vi "Motor_speed_controlling_with_PI_v7_openloop.vi"() -> ()   [LabVIEW 2016]
doc: "This example demonstrates how to generate a PWM signal on a single channel using a LINX device."
uses:
  <vilib>/MakerHub/LINX/Public/Peripherals/Analog/Analog Read 1 Chan.vi
  <vilib>/MakerHub/LINX/Public/Peripherals/Digital/Digital Read 1 Chan.vi
  <vilib>/MakerHub/LINX/Public/Peripherals/Digital/Digital Write 1 Chan.vi
  <vilib>/MakerHub/LINX/Public/Peripherals/PWM/PWM Set Duty Cycle 1 Chan.vi
  <vilib>/MakerHub/LINX/Public/Peripherals/Analog/Analog Read N Chans.vi
  <vilib>/MakerHub/LINX/Public/Peripherals/Digital/Digital Read N Chans.vi
  <vilib>/MakerHub/LINX/Public/Peripherals/Digital/Digital Write N Chans.vi
  <vilib>/MakerHub/LINX/Private/Local IO/LinxAnalogRead.vi
  <vilib>/MakerHub/LINX/Public/Utilities/Check Channel.vi
  <vilib>/MakerHub/LINX/Private/Local IO/LinxDigitalRead.vi
  <vilib>/MakerHub/LINX/Private/Local IO/LinxDigitalWrite.vi
  <vilib>/MakerHub/LINX/Public/Utilities/Open Serial.vi
  <vilib>/addons/control/pid/pid.llb/PID (DBL).vi
  <vilib>/MakerHub/LINX/Public/Peripherals/PWM/PWM Set Duty Cycle N Chans.vi
  <vilib>/MakerHub/LINX/Private/Utilties/Generate Error.vi
  <vilib>/MakerHub/LINX/LMH-LINX.lvlib
  <vilib>/addons/control/pid/NI_PID_pid.lvlib
panel:
  out "Loop Rate (Hz)":u32
  out "PWM Signal":dbl(graph)
  in  "Loop Delay(ms)":u32
  out "Motor Voltage":dbl(graph)
  out "PID Screen":dbl(graph)
  in  "Direction":bool
  out "Motor Speed(RPM)":dbl(knob) scale=0.0..80.0
  in  "Encoder Input Pin":u8
  in  "PID gains":T1={"proportional gain (Kc)"=1.0, "integral time (Ti, min)"=0.01, "derivative time (Td, min)"=0.0} {"derivative time (Td, min)" format="%.3f"; "integral time (Ti, min)" format="%.3f"; "proportional gain (Kc)" format="%.3f"}
  in  "Motor Speed":dbl(knob) scale=0.0..80.0
  in  "PWM Output Pin":u8=3
  in  "Stop Button":bool
  in  "Serial Port":refnum<visa-resource-name>
  # "Direction"
  # "Motor Speed Control\n(RPM)"
  # "Motor Speed \n(RPM)"
  # "PID Settings"
  # "Device and Connection\nSettings"
  # "Forward"
  # "e"
  # "Back"
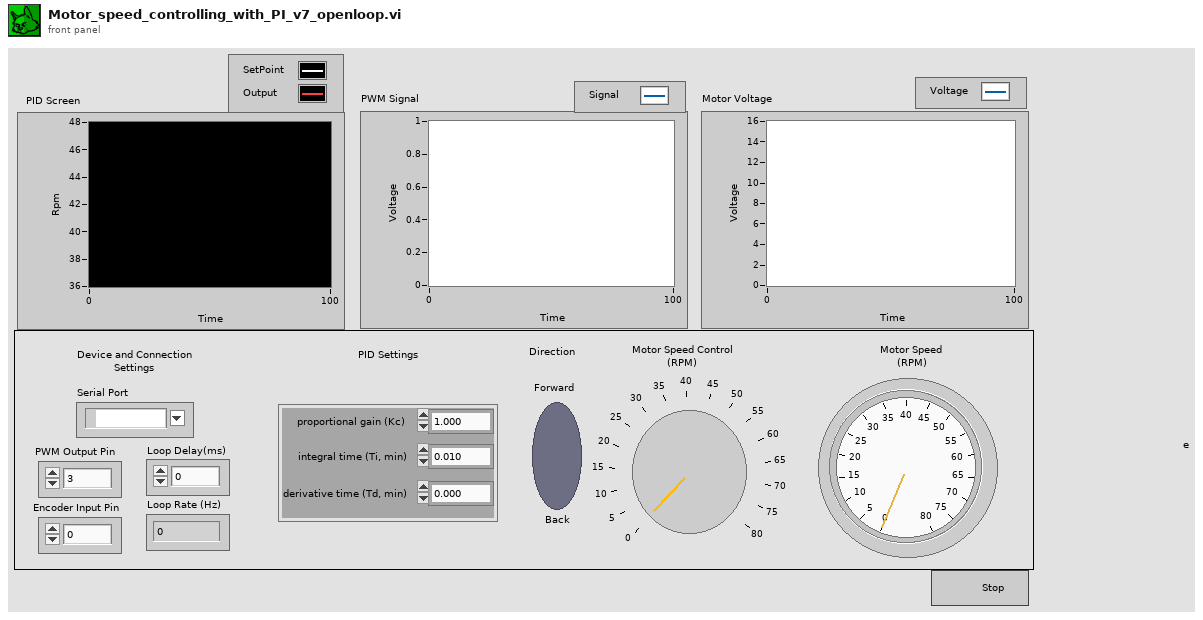
[diagram p1: front panel]
types:
  T1 = cluster{"proportional gain (Kc)":dbl, "integral time (Ti, min)":dbl, "derivative time (Td, min)":dbl}
  T2 = typedef "LMH-LINX.lvlib/LINX Ref.ctl" = cluster{"IO":T3, "Interface":T4, "LINX Device Config":T5}
  T3 = typedef "LMH-LINX.lvlib/Platform.ctl" = enum16{"Remote", "Local"}
  T4 = typedef "LMH-LINX.lvlib/Interface.ctl" = enum16{"Serial", "TCP"}
  T5 = typedef "LMH-LINX.lvlib/Device.lvlib/LINX Device Config.ctl" = cluster{"Interface":T4, "COM Port":refnum<visa-resource-name>, "TCP Configuration":T6, "Device Family":u8, "Device ID":u8, "Device Name":string, "TCP Ref":refnum<k5>, "Channels":T7}
  T6 = typedef "LMH-LINX.lvlib/Device.lvlib/TCP Config.ctl" = cluster{"IP Address":string, "Port":u16}
  T7 = typedef "LMH-LINX.lvlib/Channels.ctl" = cluster{"DI":u8[], "DO":u8[], "AI":u8[], "AO":u8[], "PWM":u8[], "QE":u8[], "UART":u8[], "I2C 2":u8[], "SPI":u8[], "CAN":u8[], "Servo":u8[], "AI Ref (V)":dbl, "AI Resolution (Bits)":u8, "AO Ref (V)":dbl, "AO Resolution (Bits)":u8}
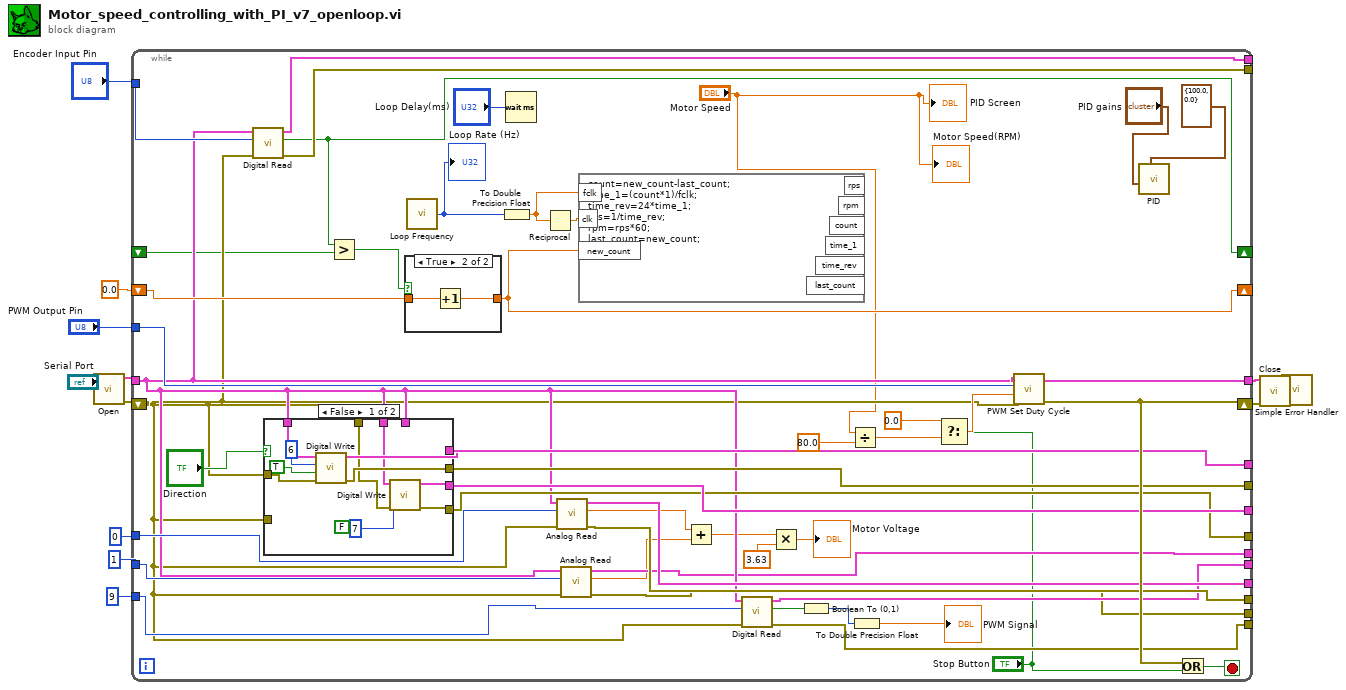
[diagram p0: block diagram]
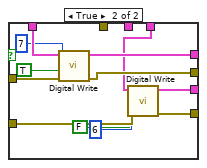
[diagram p3: hidden frame]
diagram:
  n1 = call-poly <vilib>:"Open.vi"("Serial Port"="Serial Port") -> ("Error Out"=w11:errorcluster, "LINX Resource"=w12:T2)  [unwired: 8 in, 1 out]
  n2 = while {
    tunnel: w12 -> [w29]
    tunnel: [w57] -> w10
    shift-right: [w59] -> w9
    shift-left: w11 -> [w28]
    tunnel: "PWM Output Pin" -> [w58]
    tunnel: "Encoder Input Pin" -> [w43]
    tunnel: [w42] -> _
    tunnel: [w41] -> _
    tunnel: [w51] -> _
    tunnel: [w50] -> _
    tunnel: [w47] -> _
    tunnel: [w46] -> _
    tunnel: [w45] -> _
    tunnel: [w44] -> _
    shift-right: [w16] -> _
    shift-left: _ -> [w15]
    shift-right: [w22] -> _
    shift-left: 0.0 -> [w39]
    tunnel: u8 0 ("Analog Channel") -> [w38]
    tunnel: [w37] -> _
    tunnel: [w36] -> _
    tunnel: u8 9 ("Analog Channel") -> [w33]
    tunnel: u8 1 ("Analog Channel") -> [w30]
    tunnel: [w27] -> _
    tunnel: [w26] -> _
    stop <- w60 stop-if-true
    n3 = call-poly <vilib>:"Digital Read.vi"("Error In"=w28, "DI Channel"=w43, "LINX Resource"=w29) -> ("Error Out"=w41:errorcluster, "DI Value"=w16:bool, "LINX Resource"=w42:T2)  [unwired: 6 in]
    n4 = case shown="False" "Direction" {
      tunnel: w29 -> [w75 w87]
      tunnel: w28 -> [w74 w86]
      tunnel: [w73 w84] -> w51
      tunnel: [w72 w83] -> w50
      tunnel: w29 -> [_ w81]
      tunnel: w28 -> [_ w80]
      tunnel: [w67 w79] -> w45
      tunnel: [w66 w78] -> w44
      tunnel: w29 -> [w69 _]
      tunnel: w28 -> [w68 _]
      frame False {
        n5 = call-poly <vilib>:"Digital Write.vi"("Error In"=w74, "Output Value"=TRUE, "DO Channel"=u8 6, "LINX Resource"=w75) -> ("Error Out"=w72:errorcluster, "LINX Resource"=w73:T2)  [unwired: 6 in]
        n6 = call-poly <vilib>:"Digital Write.vi"("Error In"=w68, "Output Value"=FALSE, "DO Channel"=u8 7, "LINX Resource"=w69) -> ("Error Out"=w66:errorcluster, "LINX Resource"=w67:T2)  [unwired: 6 in]
      }
      frame True {
        n7 = call-poly <vilib>:"Digital Write.vi"("Error In"=w86, "Output Value"=TRUE, "DO Channel"=u8 7, "LINX Resource"=w87) -> ("Error Out"=w83:errorcluster, "LINX Resource"=w84:T2)  [unwired: 6 in]
        n8 = call-poly <vilib>:"Digital Write.vi"("Error In"=w80, "Output Value"=FALSE, "DO Channel"=u8 6, "LINX Resource"=w81) -> ("Error Out"=w78:errorcluster, "LINX Resource"=w79:T2)  [unwired: 6 in]
      }
    }
    n9 = Greater?(x=w16, y=w15) -> (0:w14:bool)
    n10 = case shown="True" w14 {
      tunnel: w39 -> [w61 w63]
      tunnel: [w61 w62] -> w22
      frame False {
      }
      frame True {
        n11 = Increment(x=w63) -> (x+1=w62:dbl)
      }
    }
    n12 = call <vilib>:"Loop Frequency.vi"() -> ("Loop Rate (Hz)"=w21:u32)
    "Loop Rate (Hz)" <- w21
    n13 = To Double Precision Float(number=w21) -> (double precision float=w19:dbl)
    n14 = Wait (ms)(milliseconds to wait="Loop Delay(ms)") -> ()  [unwired: 1 out]
    n15 = Reciprocal(x=w19) -> (1/x=w18:dbl)
    n16 = call-poly <vilib>:"Analog Read.vi"("Error In"=w28, "Analog Channel"=w38, "LINX Resource"=w29) -> ("Error Out"=w46:errorcluster, "Voltage"=w25:dbl, "LINX Resource"=w47:T2)  [unwired: 5 in, 1 out]
    n17 = call-poly <vilib>:"Analog Read.vi"("Error In"=w28, "Analog Channel"=w30, "LINX Resource"=w29) -> ("Error Out"=w26:errorcluster, "Voltage"=w24:dbl, "LINX Resource"=w27:T2)  [unwired: 5 in, 1 out]
    n18 = formula code="count=new_count-last_count;\ntime_1=(count*1)/fclk;\ntime_rev=24*time_1;\nrps=1/time_rev;\nrpm=rps*60;\nlast_count=new_count;"("new_count"=w22, "fclk"=w19, "clk"=w18) -> ()  [unwired: 6 out]
    n19 = Add(x=w25, y=w24) -> (x+y=w23:dbl)
    n20 = call-poly <vilib>:"Digital Read.vi"("Error In"=w28, "DI Channel"=w33, "LINX Resource"=w29) -> ("Error Out"=w36:errorcluster, "DI Value"=w20:bool, "LINX Resource"=w37:T2)  [unwired: 6 in]
    n21 = Multiply(x=w23, y=3.63) -> (x*y=→"Motor Voltage":dbl)
    n22 = Boolean To (0,1)(Boolean=w20) -> (0, 1=w35:i16)
    n23 = Divide(x="Motor Speed", y=80.0) -> (x/y=w49:dbl)
    n24 = To Double Precision Float(number=w35) -> (double precision float=→"PWM Signal":dbl)
    n25 = Select(t=0.0, s="Stop Button", f=w49) -> (s? t:f=w53:dbl)
    n26 = call-poly <vilib>:"PWM Set Duty Cycle.vi"("Error In"=w28, "Duty Cycle (0-1)"=w53, "PWM Channel"=w58, "LINX Resource"=w29) -> ("Error Out"=w59:errorcluster, "LINX Resource"=w57:T2)  [unwired: 6 in]
    n27 = call-poly <vilib>:"PID.vi"("output range"=cluster{"output high":dbl, "output low":dbl} {"output high"=100.0, "output low"=0.0}, "PID gains"="PID gains") -> ()  [unwired: 8 in, 2 out]
    n28 = Or(x=w59, y="Stop Button") -> (x .or. y?=w60:bool)
    "PID Screen" <- "Motor Speed"
    "Motor Speed(RPM)" <- "Motor Speed"
  }
  n29 = call <vilib>:"Close.vi"("Error In"=w9, "LINX Resource"=w10) -> ("Error Out"=w7:errorcluster)  [unwired: 9 in]
  n30 = call <vilib>:"Simple Error Handler.vi"("error in (no error)"=w7) -> ()  [unwired: 4 in, 5 out]
